vi "Bad_position.vi"() -> ()   [LabVIEW 2020]
doc: "Przechowuje informacjê czy pojazd znajduje siê na w³aœciwej pozycji."
panel:
  in  "Boolean":bool
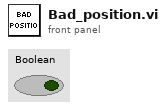
[diagram p1: front panel]
diagram:
